vi "FTW-DevUtil-XNode-SetProperties.vi"() -> ()   [LabVIEW 2015]
uses:
  <vilib>/Utility/miscctls.llb/LVPointTypeDef.ctl
panel:
  in  "Operation":bool
  in  "LazyLoad":bool
  in  "DoNotCacheAutotoolRegions":bool
  in  "Supports Fatal Error Out":bool
  in  "Style Name":string
  in  "Initial Drop Size":T1
  in  "Initial Drop Image":picture
  in  "Declared Leak Proof":bool
  in  "Version":T2
  in  "Help:Document Tag":string
  in  "Help:Document Path":path
  out "error":errorcluster
  in  "XNode Filepath":path
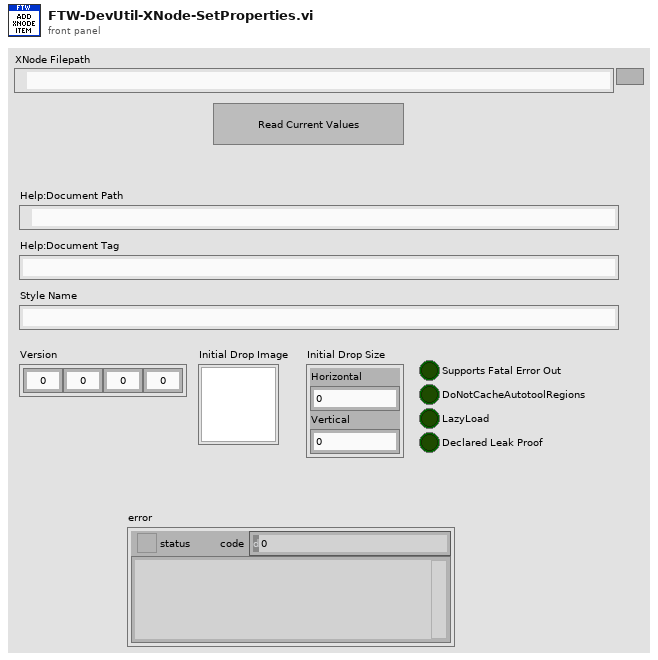
[diagram p1: front panel]
types:
  T1 = typedef "LVPointTypeDef.ctl" = cluster{"Horizontal":i16, "Vertical":i16}
  T2 = cluster{"Major":u16, "Minor":u16, "Fix":u16, "Build":u16}
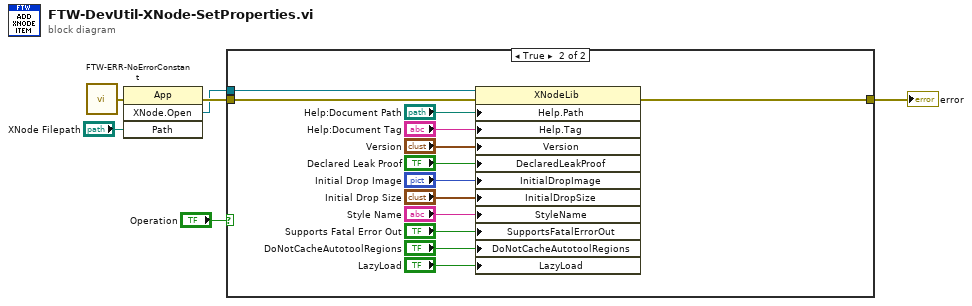
[diagram p0: block diagram]
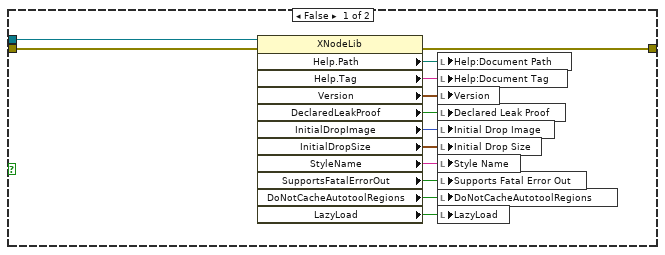
[diagram p2: hidden frame]
diagram:
  n1 = call "FTW-ERR-NoErrorConstant.vi"() -> ("no error"=w5:errorcluster)
  n2 = invoke class="App" method="XNode.Open"(error in=w5, "Path"="XNode Filepath") -> (error out=w4:errorcluster, "Open XNode"=w3:refnum<vi>)  [unwired: 2 in, 2 out]
  n3 = case shown="True" "Operation" {
    tunnel: w4 -> [w19 w32]
    tunnel: w3 -> [w18 w31]
    tunnel: [w17 w30] -> w2
    frame False {
      n4 = property class="XNodeLib"(reference=w18, error in=w19) -> (error out=w17:errorcluster, "Help.Path"=w13:path, "Help.Tag"=w14:string, "Version"=w15:T2, "DeclaredLeakProof"=w16:bool, "InitialDropImage"=w7:picture, "InitialDropSize"=w8:T1, "StyleName"=w9:string, "SupportsFatalErrorOut"=w10:bool, "DoNotCacheAutotoolRegions"=w11:bool, "LazyLoad"=w12:bool)  [unwired: 1 out]
      n5 = local write "Help:Document Path"(w13) -> ()
      n6 = local write "Help:Document Tag"(w14) -> ()
      n7 = local write "Version"(w15) -> ()
      n8 = local write "Declared Leak Proof"(w16) -> ()
      n9 = local write "Initial Drop Image"(w7) -> ()
      n10 = local write "Initial Drop Size"(w8) -> ()
      n11 = local write "Style Name"(w9) -> ()
      n12 = local write "Supports Fatal Error Out"(w10) -> ()
      n13 = local write "DoNotCacheAutotoolRegions"(w11) -> ()
      n14 = local write "LazyLoad"(w12) -> ()
    }
    frame True {
      n15 = property class="XNodeLib"(reference=w31, error in=w32, "Help.Path"="Help:Document Path", "Help.Tag"="Help:Document Tag", "Version"="Version", "DeclaredLeakProof"="Declared Leak Proof", "InitialDropImage"="Initial Drop Image", "InitialDropSize"="Initial Drop Size", "StyleName"="Style Name", "SupportsFatalErrorOut"="Supports Fatal Error Out", "DoNotCacheAutotoolRegions"="DoNotCacheAutotoolRegions", "LazyLoad"="LazyLoad") -> (error out=w30:errorcluster)  [unwired: 1 out]
    }
  }
  "error" <- w2
